vi "Meas Proc QWTB Load Result Spectra.vi"(7 "phase ref":refnum<vi>, 8 "error in":errorcluster, 11 "meas root":path) -> (0 "error out":errorcluster, 3 "graphs":T1[](array[typedef]))   [LabVIEW 2020]
uses:
  Meas Proc QWTB Spectrum Data.ctl
  other/infolib/GetString.vi
  other/infolib/Get 1D String.vi
  other/infolib/GetI64.vi
  other/infolib/Get 2D String.vi
  other/infolib/infolib.lvlib
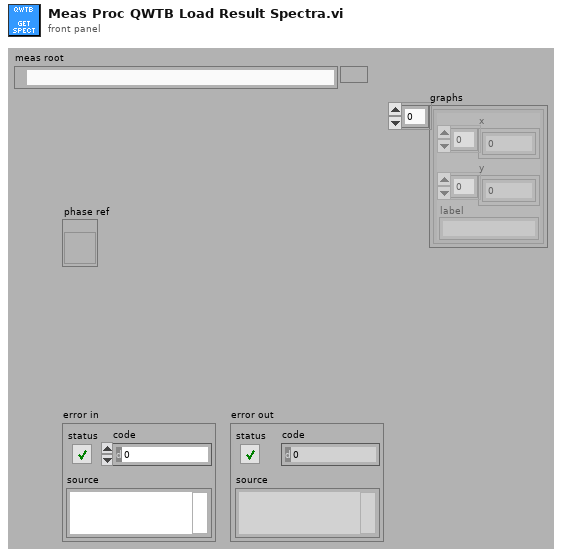
[diagram p1: front panel]
types:
  T1 = typedef "Meas Proc QWTB Spectrum Data.ctl" = cluster{"x":sgl[], "y":sgl[], "label":string}
  T2 = typedef "MAT Type Representation.ctl" = enum16{"DBL", "SGL", "I32", "I16", "U16", "U8", "CDB", "CSG", "STR"}
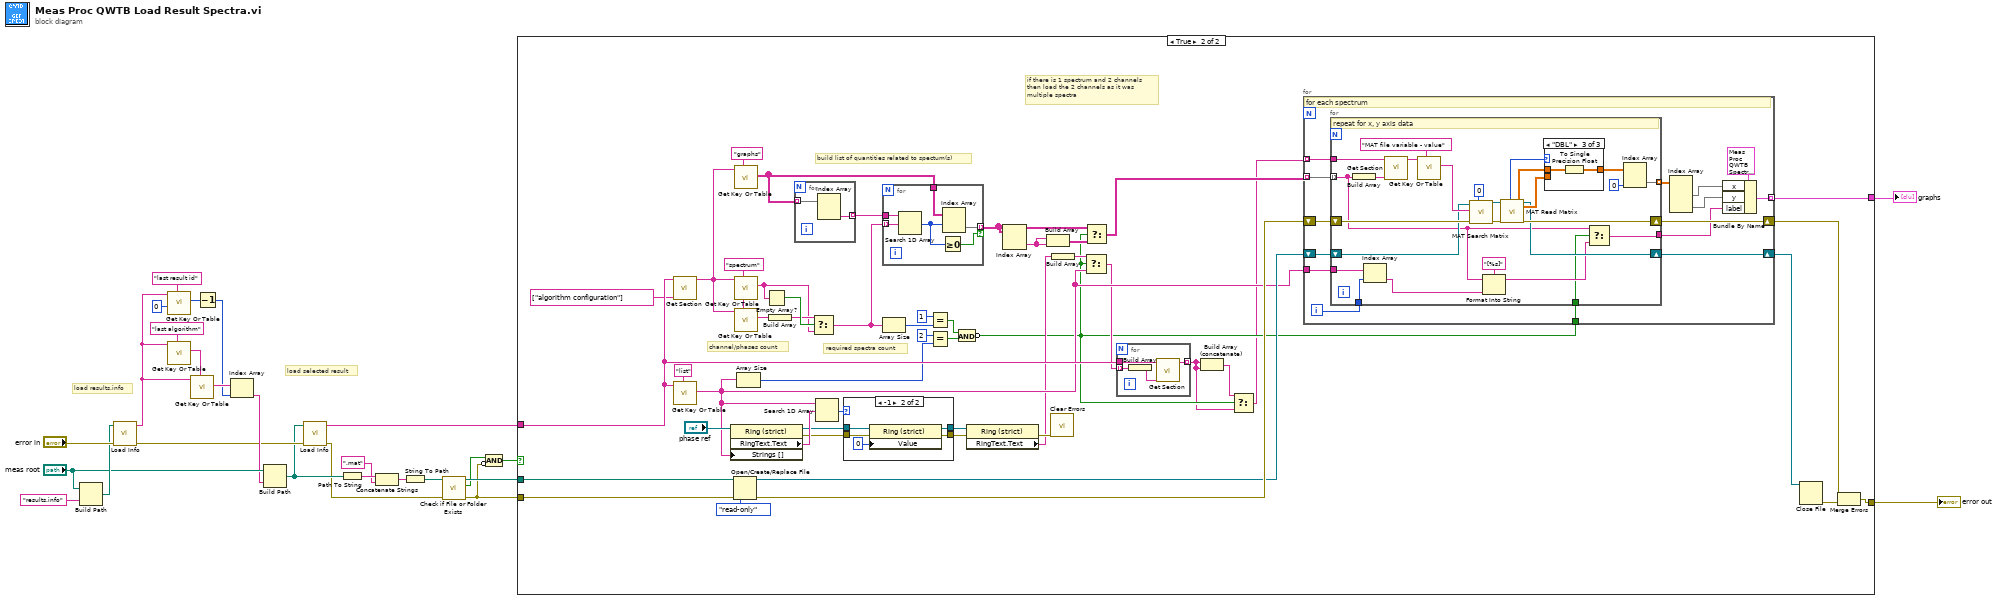
[diagram p0: block diagram]
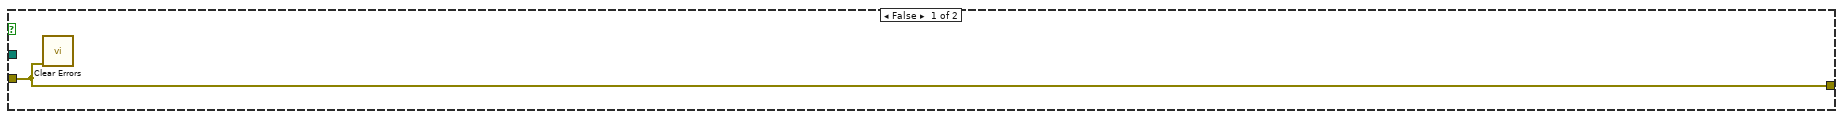
[diagram p2: hidden frame]
diagram:
  # "load selected result"
  # "load results.info"
  n1 = Build Path(base path="meas root", name or relative path="results.info") -> (appended path=w18:path)
  n2 = call "Load Info.vi"("error in"="error in", "filename"=w18) -> ("error out"=w15:errorcluster, "info data"=w23:string)  [unwired: 8 in]
  n3 = call-poly "Get Key Or Table.vi"("key description"="last result id", "numeric"=i64 0, "info data"=w23) -> ("value"=w21:i64)  [unwired: 5 in, 3 out]
  n4 = call-poly "Get Key Or Table.vi"("key description"="last algorithm", "info data"=w23) -> ("value"=w24:string)  [unwired: 6 in, 3 out]
  n5 = call-poly "Get Key Or Table.vi"("key description"=w24, "info data"=w23) -> ("value"=w22:string[])  [unwired: 6 in, 3 out]
  n6 = Decrement(x=w21) -> (x-1=w20:i64)
  n7 = Index Array(array=w22, index=w20) -> (element=w16:string)
  n8 = Build Path(base path="meas root", name or relative path=w16) -> (appended path=w12:path)
  n9 = call "Load Info.vi"("error in"=w15, "filename"=w12) -> ("error out"=w7:errorcluster, "info data"=w13:string)  [unwired: 8 in]
  n10 = Path To String(path=w12) -> (string=w11:string)
  n11 = Concatenate Strings(w11, ".mat" ("name or relative path")) -> (w9:string)
  n12 = String To Path(string=w9) -> (path=w6:path)
  n13 = call <vilib>:"Check if File or Folder Exists.vi"("error in (no error)"=w7, "path"=w6) -> ("error out"=w4:errorcluster, "file or folder exists?"=w3:bool, "dup path"=w5:path)  [unwired: 7 in]
  n14 = Compound Arithmetic op=AND(w3, invert w4) -> (w2:bool)
  n15 = case shown="True" w2 {
    tunnel: w13 -> [_ w67]
    tunnel: [_ w62] -> w8
    tunnel: [w28 w29] -> w1
    tunnel: w5 -> [_ w33]
    tunnel: w4 -> [w28 w32]
    frame False {
      n16 = call <vilib>:"Clear Errors.vi"("error in (no error)"=w28) -> ()  [unwired: 5 in, 2 out]
    }
    frame True {
      w59 = "spectrum" ("key description")
      # "if there is 1 spectrum and 2 channels\nthen load the 2 channels as it was\nmultiple spectra"
      # "channel/phases count"
      # "required spectra count"
      # "build list of quantities related to spectum(s)"
      n17 = call "Get Section.vi"("sections"=string[] ["algorithm configuration"], "info data"=w67) -> ("section part"=w58:string)  [unwired: 7 in, 2 out]
      n18 = call-poly "Get Key Or Table.vi"("key description"="list", "info data"=w67) -> ("value"=w42:string[])  [unwired: 6 in, 3 out]
      n19 = property class="Ring (strict)"(reference="phase ref", "Strings []"=w42) -> (reference out=w72:refnum<vi>, error out=w71:errorcluster, "RingText.Text"=w74:string)  [unwired: 1 in]
      n20 = Open/Create/Replace File(file path (use dialog)=w33, error in=w32, access (0:read/write)=enum16{"read/write", "read-only", "write-only"}."read-only") -> (refnum out=w61:refnum<file>, error out=w63:errorcluster)  [unwired: 3 in, 1 out]
      n21 = call-poly "Get Key Or Table.vi"("key description"="graphs", "info data"=w58) -> ("value"=w65:string[][])  [unwired: 6 in, 3 out]
      n22 = call-poly "Get Key Or Table.vi"("key description"=w59, "info data"=w58) -> ("value"=w54:string[])  [unwired: 6 in, 3 out]
      n23 = call-poly "Get Key Or Table.vi"("key description"=w59, "info data"=w58) -> ("value"=w56:string)  [unwired: 6 in, 3 out]
      n24 = Array Size(array=w42) -> (size(s)=w52:i32)
      n25 = Empty Array?(array=w54) -> (empty?=w57:bool)
      n26 = Build Array(w56) -> (w55:string[])
      n27 = for {
        tunnel: w65 -> [w89] mode=indexing
        tunnel: [w88] -> w66 mode=indexing
        n28 = Index Array(array=w89) -> (element #2=w88:string)  [unwired: 2 in, 1 out]
      }
      n29 = Select(t=w55, s=w57, f=w54) -> (s? t:f=w53:string[])
      n30 = Search 1D Array(1D array=w42, element=w74) -> (index of element=w73:i32)  [unwired: 1 in]
      n31 = case shown="-1" w73 {
        tunnel: w72 -> [w135 w140]
        tunnel: w71 -> [w134 w138]
        tunnel: [w134 w137] -> w70
        tunnel: [w135 w136] -> w69
        frame Default {
        }
        frame -1 {
          n32 = property class="Ring (strict)"(reference=w140, error in=w138, "Value"=u16 0) -> (reference out=w136:refnum<vi>, error out=w137:errorcluster)
        }
      }
      n33 = for {
        tunnel: w53 -> [w86] mode=indexing
        tunnel: w66 -> [w87]
        tunnel: w65 -> [w85]
        tunnel: [w84] -> w43 mode=indexing if=w83
        n34 = Search 1D Array(1D array=w87, element=w86) -> (index of element=w82:i32)  [unwired: 1 in]
        n35 = Greater Or Equal To 0?(x=w82) -> (x >= 0?=w83:bool)
        n36 = Index Array(array=w85, index (row)=w82) -> (element=w84:string[])  [unwired: 1 in]
      }
      n37 = Array Size(array=w53) -> (size(s)=w50:i32)
      n38 = Equal?(x=1, y=w50) -> (x = y?=w47:bool)
      n39 = Equal?(x=2, y=w52) -> (x = y?=w48:bool)
      n40 = Compound Arithmetic op=AND(w47, w48) -> (invert w38:bool)
      n41 = property class="Ring (strict)"(reference=w69, error in=w70) -> (error out=w68:errorcluster, "RingText.Text"=w41:string)  [unwired: 1 out]
      n42 = Index Array(array=w43) -> (element=w44:string[])  [unwired: 2 in]
      n43 = Build Array(w44, w44) -> (w46:string[][])
      n44 = call <vilib>:"Clear Errors.vi"("error in (no error)"=w68) -> ()  [unwired: 5 in, 2 out]
      n45 = Build Array(w41) -> (w40:string[])
      n46 = Select(t=w40, s=w38, f=w42) -> (s? t:f=w39:string[])
      n47 = Select(t=w43, s=w38, f=w46) -> (s? t:f=w45:string[][])
      n48 = for {
        tunnel: w39 -> [w81] mode=indexing
        tunnel: w67 -> [w80]
        tunnel: [w79] -> w36 mode=indexing
        n49 = Build Array(w81) -> (w78:string[])
        n50 = call "Get Section.vi"("sections"=w78, "info data"=w80) -> ("section part"=w79:string)  [unwired: 7 in, 2 out]
      }
      n51 = Build Array (concatenate)(w36, w36) -> (w37:string[])
      n52 = Select(t=w37, s=w38, f=w36) -> (s? t:f=w35:string[])
      n53 = for {
        tunnel: w45 -> [w104] mode=indexing
        tunnel: w35 -> [w103] mode=indexing
        shift-right: [w102] -> w31
        shift-left: w63 -> [w101]
        tunnel: [w97] -> w62 mode=indexing
        shift-right: [w93] -> w60
        shift-left: w61 -> [w94]
        tunnel: w42 -> [w91]
        tunnel: w38 -> [w90]
        i -> [w92]
        # "for each spectrum"
        n54 = for {
          tunnel: w104 -> [w107] mode=indexing
          tunnel: w103 -> [w130]
          shift-right: [w123] -> w102
          shift-left: w101 -> [w122]
          tunnel: [w116] -> w100 mode=indexing
          tunnel: [w113] -> w95
          shift-right: [w114] -> w93
          shift-left: w94 -> [w115]
          tunnel: w92 -> [w110]
          tunnel: w91 -> [w109]
          tunnel: w90 -> [w106]
          # "repeat for x, y axis data"
          n55 = Build Array(w107) -> (w105:string[])
          n56 = Index Array(array=w109, index=w110) -> (element=w108:string)
          n57 = call "Get Section.vi"("sections"=w105, "info data"=w130) -> ("section part"=w129:string)  [unwired: 7 in, 2 out]
          n58 = call-poly "Get Key Or Table.vi"("key description"="MAT file variable - value", "info data"=w129) -> ("value"=w127:string)  [unwired: 6 in, 3 out]
          n59 = call "MAT Search Matrix.vi"("offset in (-1: current position)"=i64 0, "Error In"=w122, "matrix name"=w127, "Ref Num"=w115) -> ("error out"=w125:errorcluster, "Dup Ref Num"=w124:refnum<file>)  [unwired: 6 in]
          n60 = Format Into String(format string="[%s]", initial string=w107, w108) -> (resulting string=w111:string)  [unwired: 1 in, 1 out]
          n61 = call "MAT Read Matrix.vi"("Ref Num"=w124, "Error In"=w125) -> ("Representation"=w121:T2, "DBL"=w119:dbl[][], "Dup Ref Num"=w114:refnum<file>, "SGL"=w120:sgl[][], "error out"=w123:errorcluster)  [unwired: 5 in, 8 out]
          n62 = case shown="\"DBL\"" w121 {
            tunnel: w120 -> [w131 _ _]
            tunnel: w119 -> [_ _ w133]
            tunnel: [w131 _ w132] -> w118
            frame "SGL" {
            }
            frame Default {
            }
            frame "DBL" {
              n63 = To Single Precision Float(number=w133) -> (single precision float=w132:sgl[][])
            }
          }
          n64 = Select(t=w107, s=w106, f=w111) -> (s? t:f=w113:string)
          n65 = Index Array(array=w118, index (col)=0 ("disabled index (col)")) -> (element=w116:sgl[])  [unwired: 1 in]
        }
        n66 = Index Array(array=w100) -> (element #1=w99:sgl[], element #2=w98:sgl[])  [unwired: 4 in]
        n67 = Bundle By Name(cluster=T1 {"x"=array[24001 elements], "y"=array[24001 elements], "label"=""} ("Meas Proc QWTB Spectrum Data"), "x"=w99, "y"=w98, "label"=w95) -> (w97:T1)
      }
      n68 = Close File(refnum=w60) -> (error out=w30:errorcluster)  [unwired: 1 in, 1 out]
      n69 = Merge Errors(w31, w30) -> (w29:errorcluster)
    }
  }
  "error out" <- w1
  "graphs" <- w8
